vi "TruncSGL.vi"(5 "Decimal places":i8, 6 "Number":sgl format="%#.10f") -> (2 "Truncated number":sgl format="%#.10f")   [LabVIEW 2017, in "GPNumeric.lvlib"]
doc: "Truncates <B>Number</B> to a number of <B>Decimal places</B>.\n\nYou can set <B>Decimal places</B> to a negative number to truncate to nearest 10, nearest 100 and so on. E.g. to truncate 782.402 to the nearest hundred, you set <B>Decimal places</B> to -2 and the <B>Truncated number</B> will be 700.\n\nThis VI is inlined.\n\nSteen Schmidt\nGPower\n5/4 2014"
uses:
  GPNumeric.lvlib
panel:
  # "Copyright © 2014\nGPower\nSee enclosed license file for terms and conditions"
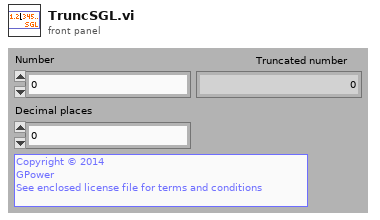
[diagram p1: front panel]
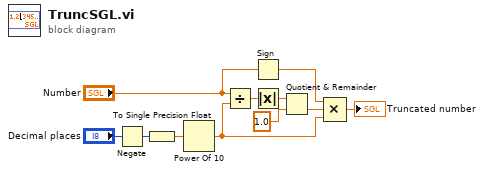
[diagram p0: block diagram]
diagram:
  n1 = Negate(x="Decimal places") -> (-x=w11:i8)
  n2 = To Single Precision Float(number=w11) -> (single precision float=w1:sgl)
  n3 = Power Of 10(x=w1) -> (10^x=w5:sgl)
  n4 = Divide(x="Number", y=w5) -> (x/y=w10:sgl)
  n5 = Sign(1:"Number") -> (0:w3:sgl)
  n6 = Absolute Value(x=w10) -> (abs(x)=w7:sgl)
  n7 = Quotient & Remainder(x=w7, y=sgl 1.0) -> (floor(x/y)=w4:sgl)  [unwired: 1 out]
  n8 = Compound Arithmetic op=MULTIPLY(w3, w4, w5) -> (→"Truncated number":sgl)
